vi "test Duplicate.vi"(8 "error in (no error)":errorcluster, 11 "TestCase In":refnum<class "Data Manipulation Tests.lvclass">) -> (0 "error out":errorcluster, 3 "TestCase Out":refnum<class "Data Manipulation Tests.lvclass">)   [LabVIEW 2017, in "Pointer Tests.lvlib" / "Data Manipulation Tests.lvclass"]
uses:
  Data Manipulation Tests.lvclass
  <vilib>/addons/_JKI Toolkits/VI Tester/TestCase.llb/TestCase.lvclass
  Source/Classes/Pointer/Pointer.lvclass
  Source/Classes/Pointer/Write 1D I32.vi
  C:/Program Files (x86)/National Instruments/LabVIEW 2017/vi.lib/addons/_JKI Toolkits/VI Tester/TestCase.llb/TestCase.lvclass
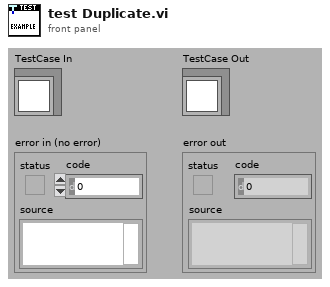
[diagram p1: front panel]
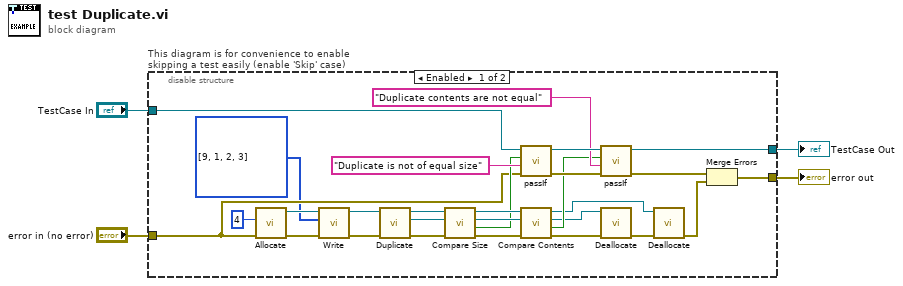
[diagram p0: block diagram]
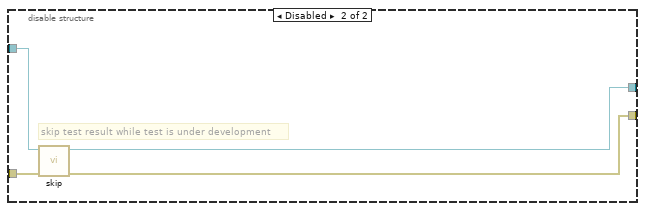
[diagram p2: hidden frame]
diagram:
  n1 = disable-structure "This diagram is for convenience to enable skipping a test easily (enable 'Skip' case)" shown="Enabled" {
    disable-tunnel: "TestCase In" -> [w30 w36]
    disable-tunnel: [w27 w34] -> w1
    disable-tunnel: [w12 w35] -> w3
    disable-tunnel: "error in (no error)" -> [w10 w33]
    frame Enabled {
      n2 = call "Allocate.vi"("error in (no error)"=w10, "size"=u64 4 ("count (1)")) -> ("error out"=w15:errorcluster, "Pointer out"=w32:refnum<class "Pointer.lvclass">)  [unwired: 8 in]
      n3 = call-poly "Write.vi"("error in (no error)"=w15, "buffer in"=i32[] [9, 1, 2, 3] ("count (1)"), "Pointer in"=w32) -> ("error out"=w14:errorcluster, "Pointer out"=w16:refnum<class "Pointer.lvclass">)  [unwired: 5 in, 2 out]
      n4 = call "Duplicate.vi"("error in (no error)"=w14, "Pointer in"=w16) -> ("error out"=w23:errorcluster, "new Pointer"=w20:refnum<class "Pointer.lvclass">, "Pointer out"=w24:refnum<class "Pointer.lvclass">)  [unwired: 7 in]
      n5 = call "Compare Size.vi"("error in (no error)"=w23, "Pointer b in"=w20, "Pointer a in"=w24) -> ("error out"=w21:errorcluster, "equal size?"=w18:bool, "Pointer b out"=w19:refnum<class "Pointer.lvclass">, "Pointer a out"=w22:refnum<class "Pointer.lvclass">)  [unwired: 5 in]
      n6 = call-dynamic "passIf.vi"("error in (no error)"=w10, "message (\"\")"="Duplicate is not of equal size" ("message (\"\")"), "pass"=w18, "TestCase in"=w30) -> ("error out"=w31:errorcluster, "TestCase out"=w28:refnum<class "Data Manipulation Tests.lvclass">)  [unwired: 6 in]
      n7 = call "Compare Contents.vi"("error in (no error)"=w21, "Pointer b in"=w19, "Pointer a in"=w22) -> ("error out"=w11:errorcluster, "equal contents?"=w17:bool, "Pointer b out"=w7:refnum<class "Pointer.lvclass">, "Pointer a out"=w6:refnum<class "Pointer.lvclass">)  [unwired: 5 in]
      n8 = call-dynamic "passIf.vi"("error in (no error)"=w31, "message (\"\")"="Duplicate contents are not equal" ("message (\"\")"), "pass"=w17, "TestCase in"=w28) -> ("error out"=w29:errorcluster, "TestCase out"=w27:refnum<class "Data Manipulation Tests.lvclass">)  [unwired: 6 in]
      n9 = call "Deallocate.vi"("error in (no error)"=w11, "Pointer in"=w7) -> ("error out"=w9:errorcluster)  [unwired: 8 in, 1 out]
      n10 = call "Deallocate.vi"("error in (no error)"=w9, "Pointer in"=w6) -> ("error out"=w8:errorcluster)  [unwired: 8 in, 1 out]
      n11 = Merge Errors(w29, w8) -> (w12:errorcluster)
    }
    frame Disabled {
      # "skip test result while test is under development"
      n12 = call <vilib>:"skip.vi"("error in (no error)"=w33, "TestCase in"=w36) -> ("error out"=w35:errorcluster, "TestCase out"=w34:refnum<class "Data Manipulation Tests.lvclass">)  [unwired: 8 in]
    }
  }
  "error out" <- w3
  "TestCase Out" <- w1
